vi "Caller VI_Keep ApplyLib in Memory.vi"   [LabVIEW 2021]
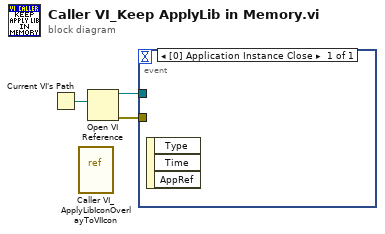
[diagram p0: block diagram]
diagram:
  n1 = Current VI's Path() -> (path=w3:path)
  n2 = vi-ref "Caller VI_ApplyLibIconOverlayToVIIcon.vi"() -> ()  [unwired: 1 out]
  n3 = Open VI Reference(vi path=w3) -> (vi reference=w1:refnum<vi>, error out=w2:errorcluster)  [unwired: 1 in, 4 out]
  n4 = event shown="[0] Application Instance Close" {
    selector: _ -> [_]
    dyn-events: _ -> [_]
    timeout: _ -> [_]
    tunnel: w2 -> [_]
    tunnel: w1 -> [_]
    event Application Instance Close {
      n5 = event-data() -> ()  [unwired: 4 out]
    }
  }
